vi "Load Tree by Table.vi"(8 "error in (no error)":errorcluster, 10 "Table":string[][](array[string]), 11 "Tree in":refnum<class "TreeControl.lvclass">) -> (0 "error out":errorcluster, 3 "Tree out":refnum<class "TreeControl.lvclass">)   [LabVIEW 2015, in "TreeControl.lvclass"]
doc: "This method will load the table data into the tree as long as the table data is ordered correctly. The data must be formatted so that:\n\n column 0 = Child Tags\n column 1 = Parent Tags\n column 2 = Left Cell String\ncolumn 3..n = Child Text[]\n<b> </b> <b> </b>\n©2016 Q Software Innovations, LLC (QSI)\nwritten by Quentin Alldredge\nproduced in LabVIEW 2015\n\nsupport@qsoftwareinnovations.com\nwww.qsoftwareinnovations.com\n\nAll rights reserved.\n\nRedistribution and use in source and binary forms, with or without modification, are permitted provided that the following conditions are met:\n\n * Redistributions of source code must retain the above copyright notice, this list of conditions and the following disclaimer.\n * Redistributions in binary form must reproduce the above copyright notice, this list of conditions and the following disclaimer in the documentation and/or other materials provided with the distribution.\n * Neither the name of Q Software Innovations, LLC. nor the names of its contributors may be used to endorse or promote products derived from this software without specific prior written permission.\n\nTHIS SOFTWARE IS PROVIDED BY THE COPYRIGHT HOLDERS AND CONTRIBUTORS \"AS IS\" AND ANY EXPRESS OR IMPLIED WARRANTIES, INCLUDING, BUT NOT LIMITED TO, THE IMPLIED WARRANTIES OF MERCHANTABILITY AND FITNESS FOR A PARTICULAR PURPOSE ARE DISCLAIMED. IN NO EVENT SHALL THE COPYRIGHT OWNER OR CONTRIBUTORS BE LIABLE FOR ANY DIRECT, INDIRECT, INCIDENTAL, SPECIAL, EXEMPLARY, OR CONSEQUENTIAL DAMAGES (INCLUDING, BUT NOT LIMITED TO, PROCUREMENT OF SUBSTITUTE GOODS OR SERVICES; LOSS OF USE, DATA, OR PROFITS; OR BUSINESS INTERRUPTION) HOWEVER CAUSED AND ON ANY THEORY OF LIABILITY, WHETHER IN CONTRACT, STRICT LIABILITY, OR TORT (INCLUDING NEGLIGENCE OR OTHERWISE) ARISING IN ANY WAY OUT OF THE USE OF THIS SOFTWARE, EVEN IF ADVISED OF THE POSSIBILITY OF SUCH DAMAGE."
uses:
  TreeControl.lvclass
  Add Item Info Cluster.ctl
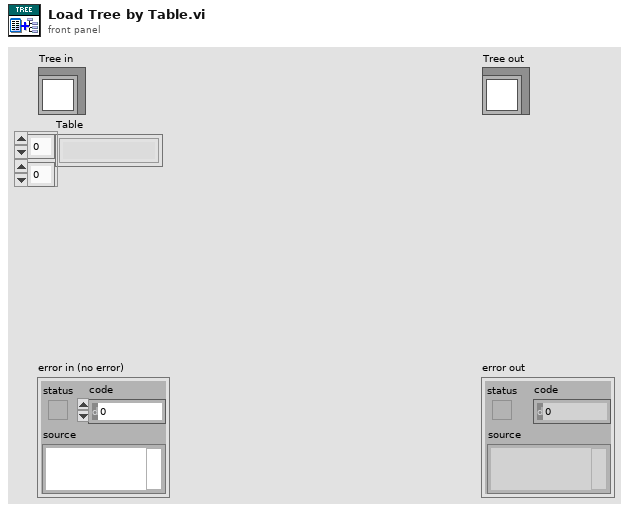
[diagram p1: front panel]
types:
  T1 = typedef "TreeControl.lvclass/Add Item Info Cluster.ctl" = cluster{"Parent Tag (\"\")":string, "Child Position (-1=End)":i32, "Left Cell String (\"\" = Same as Child Tag)":string, "Child Text[]":string[], "Child Tag":string, "Child Only? (F)":bool}
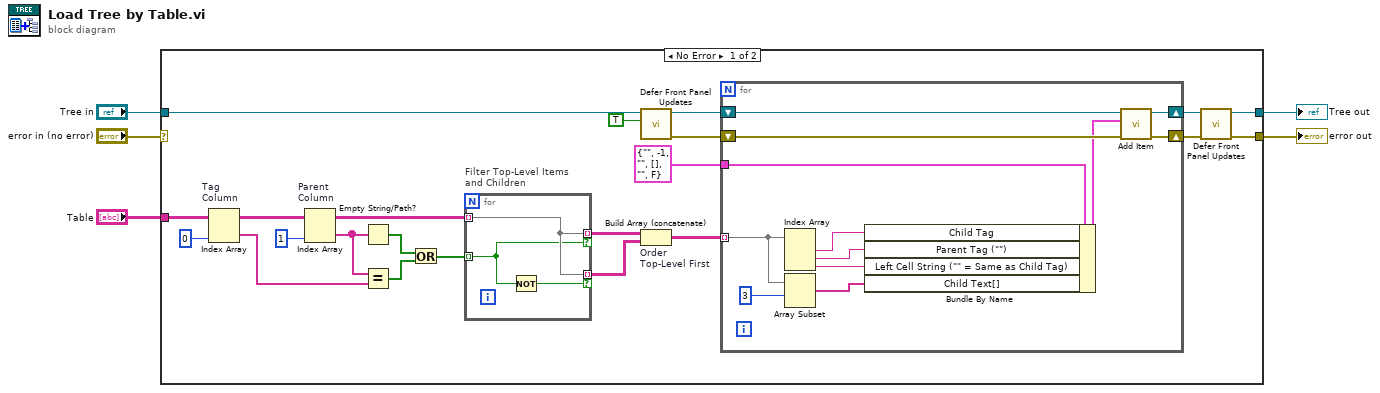
[diagram p0: block diagram]
diagram:
  n1 = case shown="No Error" "error in (no error)" {
    selector: "error in (no error)" -> [_ w42]
    tunnel: [w11 w42] -> w4
    tunnel: [w10 w41] -> w2
    tunnel: "Tree in" -> [w9 w41]
    tunnel: "Table" -> [w18 _]
    frame No Error {
      n2 = Index Array "Tag \nColumn"(array=w18, index (col)=0 ("disabled index (col)")) -> (element=w23:string[])  [unwired: 1 in]
      n3 = Index Array "Parent \nColumn"(array=w18, index (col)=1 ("disabled index (col)")) -> (element=w22:string[])  [unwired: 1 in]
      n4 = Empty String/Path?(string/path=w22) -> (empty?=w21:bool[])
      n5 = Equal?(x=w22, y=w23) -> (x = y?=w20:bool[])
      n6 = Or(x=w21, y=w20) -> (x .or. y?=w19:bool[])
      n7 = for "Filter Top-Level Items\nand Children" {
        tunnel: w19 -> [w39] mode=indexing
        tunnel: [w40] -> w16 mode=indexing if=w39
        tunnel: w18 -> [w40] mode=indexing
        tunnel: [w40] -> w15 mode=indexing if=w38
        n8 = Not(x=w39) -> (.not. x?=w38:bool)
      }
      n9 = call "Defer Front Panel Updates.vi"("Defer Panel Updates (F)"=TRUE, "Tree in"=w9) -> ("error out"=w17:errorcluster, "Tree (dup)"=w8:refnum<class "TreeControl.lvclass">)  [unwired: 8 in]
      n10 = Build Array (concatenate) "Order \nTop-Level First"(w16, w15) -> (w14:string[][])
      n11 = for {
        shift-right: [w32] -> w13
        shift-left: w17 -> [w33]
        tunnel: w14 -> [w37] mode=indexing
        shift-right: [w34] -> w7
        shift-left: w8 -> [w35]
        tunnel: T1 {"Parent Tag (\"\")"="", "Child Position (-1=End)"=-1, "Left Cell String (\"\" = Same as Child Tag)"="", "Child Text[]"=[], "Child Tag"="", "Child Only? (F)"=FALSE} ("AddItemInfo") -> [w31]
        n12 = Index Array(array=w37) -> (element #1=w30:string, element #2=w29:string, element #3=w28:string)  [unwired: 3 in]
        n13 = Array Subset(array=w37, index=3) -> (w26:string[])  [unwired: 1 in]
        n14 = Bundle By Name(cluster=w31, "Child Tag"=w30, "Parent Tag (\"\")"=w29, "Left Cell String (\"\" = Same as Child Tag)"=w28, "Child Text[]"=w26) -> (w27:T1)
        n15 = call-dynamic "Add Item.vi"("error in (no error)"=w33, "ItemInfo"=w27, "Tree in"=w35) -> ("error out"=w32:errorcluster, "Tree (dup)"=w34:refnum<class "TreeControl.lvclass">)  [unwired: 6 in, 1 out]
      }
      n16 = call "Defer Front Panel Updates.vi"("error in (no error)"=w13, "Tree in"=w7) -> ("error out"=w11:errorcluster, "Tree (dup)"=w10:refnum<class "TreeControl.lvclass">)  [unwired: 8 in]
    }
    frame Error {
    }
  }
  "error out" <- w4
  "Tree out" <- w2
